vi "Get Node Data RecursiveChild.vi"(10 "Node Path (parent, child)":string[](array[string]), 11 "Tree Map In":T3) -> (0 "error out":errorcluster, 1 "Node Exists?":bool, 2 "Node Data":T1, 3 "Tree Map Out":T3)   [LabVIEW 2020, in "Blue Tree Map OpenSource.lvlib"]
uses:
  Blue Tree Map OpenSource.lvlib
  Typedefs/Tree Map.ctl
  Typedefs/Tree Map Data.ctl
  Typedefs/Tree Node Data.ctl
  Typedefs/Attribute Map.ctl
  <vilib>/Utility/miscctls.llb/LVMapReplaceAction.ctl
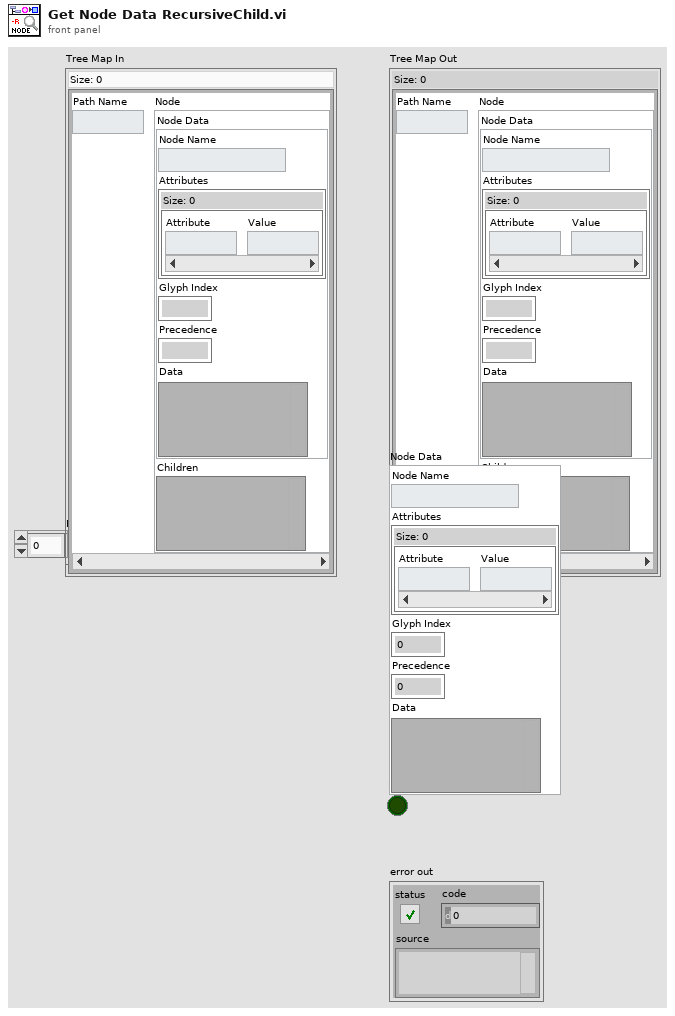
[diagram p1: front panel]
types:
  T1 = typedef "Blue Tree Map OpenSource.lvlib/Tree Node Data.ctl" = cluster{"Node Name":string, "Attributes":T2, "Glyph Index":i32, "Precedence":i32, "Data":variant}
  T2 = typedef "Blue Tree Map OpenSource.lvlib/Attribute Map.ctl" = map{string, string}
  T3 = typedef "Blue Tree Map OpenSource.lvlib/Tree Map.ctl" = map{string, T4}
  T4 = typedef "Blue Tree Map OpenSource.lvlib/Tree Map Data.ctl" = cluster{"Node Data":T1, "Children":variant}
  T5 = typedef "LVMapReplaceAction.ctl" = enum32{"Modify Entry only if found", "Add or Modify Entry", "Delete Entry"}
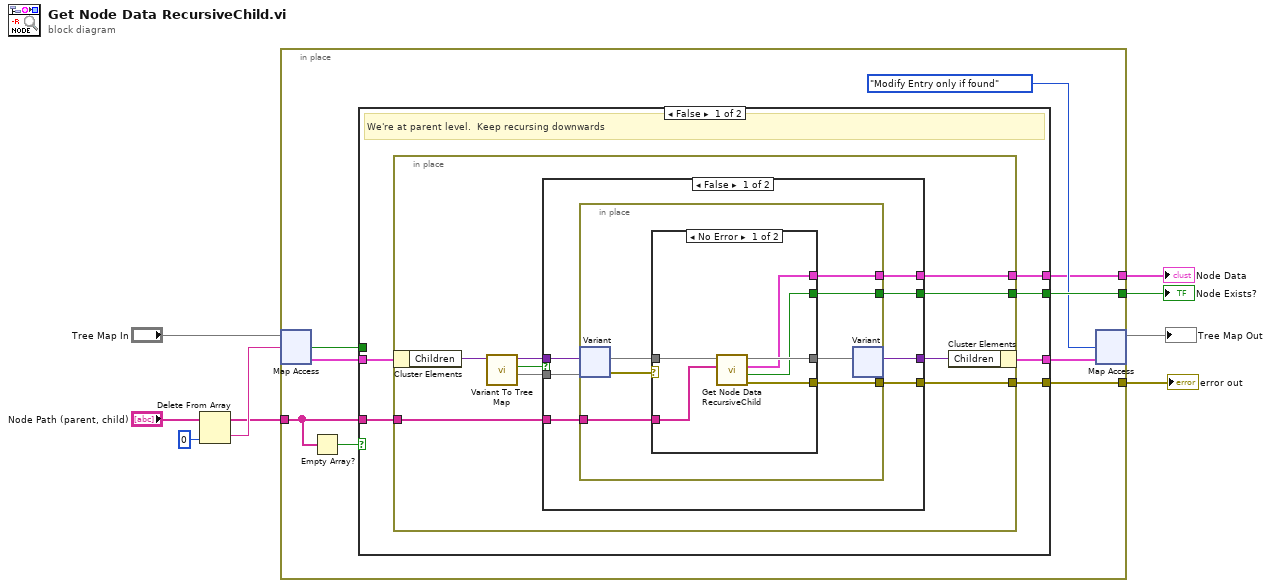
[diagram p0: block diagram]
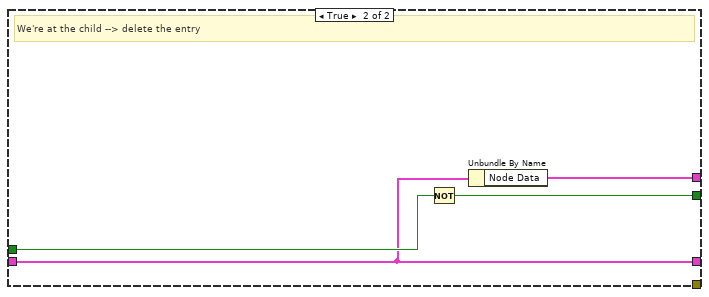
[diagram p4: hidden frame]
diagram:
  n1 = Delete From Array(array="Node Path (parent, child)", index=0) -> (deleted portion=w8:string, array with subset deleted=w7:string[])  [unwired: 1 in]
  n2 = in-place {
    in-place-border: w7 -> [w12]
    in-place-border: [w17] -> w3
    in-place-border: [w15] -> w4
    in-place-border: [w10] -> w1
    n3 = in-place-map #1("Tree Map In", w8) -> (w18:T4, w14:bool)  [unwired: 1 in]
    n4 = Empty Array?(array=w12) -> (empty?=w13:bool)
    n5 = case shown="False" w13 {
      tunnel: w18 -> [w24 w58]
      tunnel: w12 -> [w23 _]
      tunnel: [w22 _] -> w17
      tunnel: [w21 w58] -> w16
      tunnel: [w20 w60] -> w15
      tunnel: w14 -> [_ w59]
      tunnel: [w19 w57] -> w10
      frame False {
        # "We're at parent level.  Keep recursing downwards"
        n6 = in-place {
          in-place-border: w23 -> [w32]
          in-place-border: [w31] -> w22
          in-place-border: [w30] -> w20
          in-place-border: [w25] -> w19
          n7 = in-place-cluster #2(w24) -> ("Children"=w33:variant)
          n8 = call "Variant To Tree Map.vi"("Children"=w33) -> ("Tree Map (Empty)"=w28:T3, "Empty?"=w27:bool, "Children"=w29:variant)  [unwired: 8 in]
          n9 = case shown="False" w27 {
            tunnel: w32 -> [w40 _]
            tunnel: [w39 _] -> w31
            tunnel: [w38 _] -> w30
            tunnel: w29 -> [w37 w56]
            tunnel: w28 -> [w36 _]
            tunnel: [w35 w56] -> w26
            tunnel: [w34 _] -> w25
            frame False {
              n10 = in-place {
                in-place-border: w40 -> [w47]
                in-place-border: [w46] -> w39
                in-place-border: [w45] -> w38
                in-place-border: [w41] -> w34
                n11 = in-place-variant #3(w37, w36) -> (w44:T3, w42:errorcluster)
                n12 = case shown="No Error" w42 {
                  selector: w42 -> [_ w54]
                  tunnel: w47 -> [w50 _]
                  tunnel: [w51 w54] -> w46
                  tunnel: [w49 _] -> w45
                  tunnel: w44 -> [w53 w55]
                  tunnel: [w52 w55] -> w43
                  tunnel: [w48 _] -> w41
                  frame No Error {
                    n13 = call "Get Node Data RecursiveChild.vi"("Node Path (parent, child)"=w50, "Tree Map In"=w53) -> ("error out"=w51:errorcluster, "Node Exists?"=w49:bool, "Node Data"=w48:T1, "Tree Map Out"=w52:T3)  [unwired: 6 in]
                  }
                  frame Error {
                  }
                }
                n14 = in-place-variant #3(w43) -> (w35:variant)  [unwired: 1 out]
              }
            }
            frame True {
            }
          }
          n15 = in-place-cluster #2("Children"=w26) -> (w21:T4)
        }
      }
      frame True {
        # "We're at the child --> delete the entry"
        n16 = Not(x=w59) -> (.not. x?=w60:bool)
        n17 = Unbundle By Name(w58) -> ("Node Data"=w57:T1)
      }
    }
    n18 = in-place-map #1(w16, LVMapReplaceAction."Modify Entry only if found" ("action")) -> (→"Tree Map Out":T3)  [unwired: 2 out]
  }
  "error out" <- w3
  "Node Exists?" <- w4
  "Node Data" <- w1
